vi "BuildConcentrationString.vi"(1 "Concentrations":dbl[](array[numeric])) -> (0 "Concentration String":string[](array[string]))   [LabVIEW 2013]
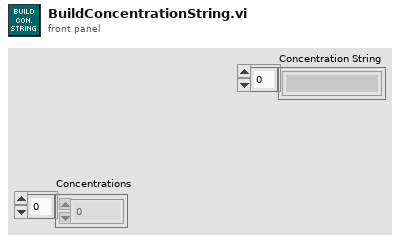
[diagram p1: front panel]
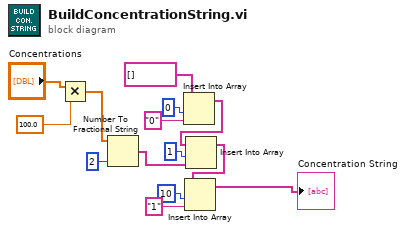
[diagram p0: block diagram]
diagram:
  n1 = Multiply(x="Concentrations", y=100.0) -> (x*y=w2:dbl[])
  n2 = Number To Fractional String(number=w2, precision (6)=i16 2) -> (F-format string=w8:string[])  [unwired: 2 in]
  n3 = Insert Into Array(array=string[] [], index=0, new element="0" ("new element/subarray")) -> (w9:string[])
  n4 = Insert Into Array(array=w9, index=1, new element=w8) -> (w5:string[])
  n5 = Insert Into Array(array=w5, index=10, new element="1" ("new element/subarray")) -> (→"Concentration String":string[])
